vi "Configure Synchronous Simultaneous Interface.vi"(6 "Slave Address (0)":i32, 8 "error in (no error)":errorcluster, 9 "Master Address":i32[](array[numeric])=[0, 1], 10 "SSI State (2: None)":u16(ring)=2 items=["Master", "Slave", "None"], 11 "VISA resource name":refnum<visa-resource-name>) -> (0 "error out":errorcluster, 3 "VISA resource name out":refnum<visa-resource-name>)   [LabVIEW 2010, in "Agilent U2722.lvlib"]
doc: "Configures the instrument's role in a chassis."
uses:
  Agilent U2722.lvlib
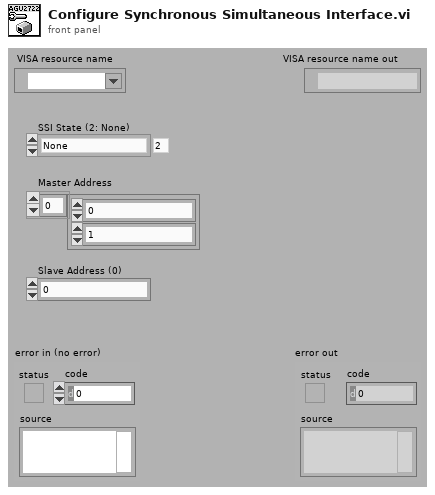
[diagram p1: front panel]
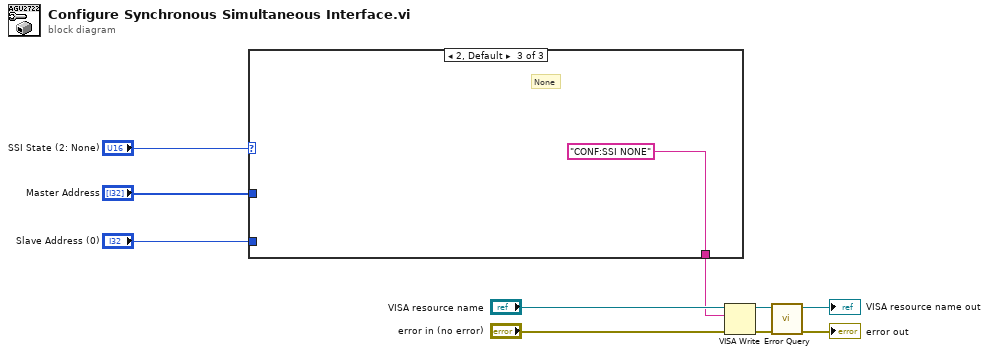
[diagram p0: block diagram]
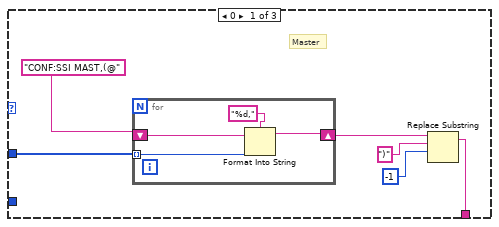
[diagram p2: hidden frame]
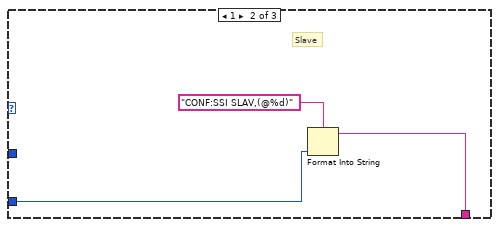
[diagram p3: hidden frame]
diagram:
  n1 = case shown="2, Default" "SSI State (2: None)" {
    tunnel: "Master Address" -> [w16 _ _]
    tunnel: [w11 w21 "CONF:SSI NONE"] -> w2
    tunnel: "Slave Address (0)" -> [_ w22 _]
    frame 0 {
      # "Master"
      n2 = for {
        tunnel: w16 -> [w20] mode=indexing
        shift-right: [w17] -> w14
        shift-left: "CONF:SSI MAST,(@" -> [w19]
        n3 = Format Into String(format string="%d," ("initial string"), initial string=w19, w20) -> (resulting string=w17:string)  [unwired: 1 in, 1 out]
      }
      n4 = Replace Substring(3:-1 ("offset (0)"), 4:")" ("substring (\"\")"), 5:w14) -> (1:w11:string)  [unwired: 1 in, 1 out]
    }
    frame 1 {
      # "Slave"
      n5 = Format Into String(format string="CONF:SSI SLAV,(@%d)", w22) -> (resulting string=w21:string)  [unwired: 2 in, 1 out]
    }
    frame 2, Default {
      # "None"
    }
  }
  n6 = VISA Write(VISA resource name="VISA resource name", write buffer=w2, error in (no error)="error in (no error)") -> (VISA resource name out=w6:refnum<visa-resource-name>, error out=w5:errorcluster)  [unwired: 1 out]
  n7 = call "Error Query.vi"("error in (no error)"=w5, "VISA resource name"=w6) -> ("error out"=→"error out":errorcluster, "VISA resource name out"=→"VISA resource name out":refnum<visa-resource-name>)  [unwired: 6 in, 2 out]
